vi "DB Tools Create Parameterized Query.vi"(4 "stored procedure? (F)":bool, 5 "auto-detect parameters? (F)":bool, 6 "error in (no error)":errorcluster, 7 "parameters":T3[](array[typedef]), 8 "SQL query":string, 9 "connection reference":T2) -> (0 "error out":errorcluster, 1 "parameters out":T3[](array[typedef]), 3 "command reference":T6)   [LabVIEW 2020, in "NI_Database_API.lvlib"]
doc: "Creates a parameterized <B>SQL query</B> and returns a <B>command reference</B> that you must free eventually. Unless you are detecting the parameters automatically, the number of elements in the <B>parameters</B> array must match the number of parameters you specify in <B>SQL query</B>. For stored procedures, set <B>stored procedure</B> to TRUE and <B>SQL query</B> to the name of the procedure you want to execute."
uses:
  <vilib>/addons/database/NI_Database_API.lvlib
  <vilib>/addons/database/Connection.llb/Conn ObjectReference.ctl
  <vilib>/addons/database/Command.llb/Cmd ObjectReference.ctl
  <vilib>/addons/database/Command.llb/Cmd DataMembers.ctl
  <vilib>/addons/database/Auxilliary.llb/DB Tools Parameter Info.ctl
  <vilib>/addons/database/Auxilliary.llb/DB Tools DataTypes.ctl
  <vilib>/addons/database/Auxilliary.llb/DB Tools Parameter Dir.ctl
  <vilib>/addons/database/Connection.llb/Conn Get Properties.vi
panel:
  in  "default":T1
  in  "default data":T1
  in  "ADODB._Command":refnum<k7>
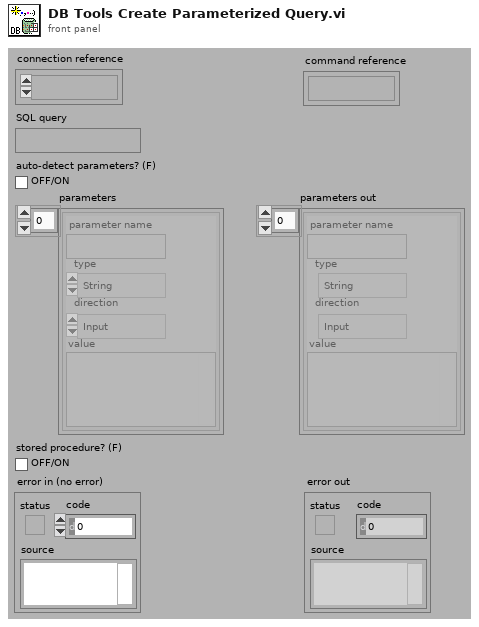
[diagram p1: front panel]
types:
  T1 = typedef "NI_Database_API.lvlib/Cmd DataMembers.ctl" = cluster{"ADODB._Command":refnum<k7>, "Connection":T2}
  T2 = typedef "NI_Database_API.lvlib/Conn ObjectReference.ctl" = refnum<k1>
  T3 = typedef "NI_Database_API.lvlib/DB Tools Parameter Info.ctl" = cluster{"parameter name":string, "type":T4, "direction":T5, "value":variant}
  T4 = typedef "NI_Database_API.lvlib/DB Tools DataTypes.ctl" = enum16{"String", "Long (I32)", "Single (SGL)", "Double (DBL)", "Date/Time", "Binary"}
  T5 = typedef "NI_Database_API.lvlib/DB Tools Parameter Dir.ctl" = enum32{"Input", "Output", "Input/Output", "Return Value"}
  T6 = typedef "NI_Database_API.lvlib/Cmd ObjectReference.ctl" = refnum<k1>
  T7 = typedef "NI_Database_API.lvlib/Conn Properties.ctl" = cluster{"command timeout (s)":i32, "connection string":string, "default database":string, "provider":string}
  T8 = typedef "NI_Database_API.lvlib/Conn DataMembers.ctl" = cluster{"ADODB._Connection":refnum<k7>, "recordset objects":i32, "command objects":i32}
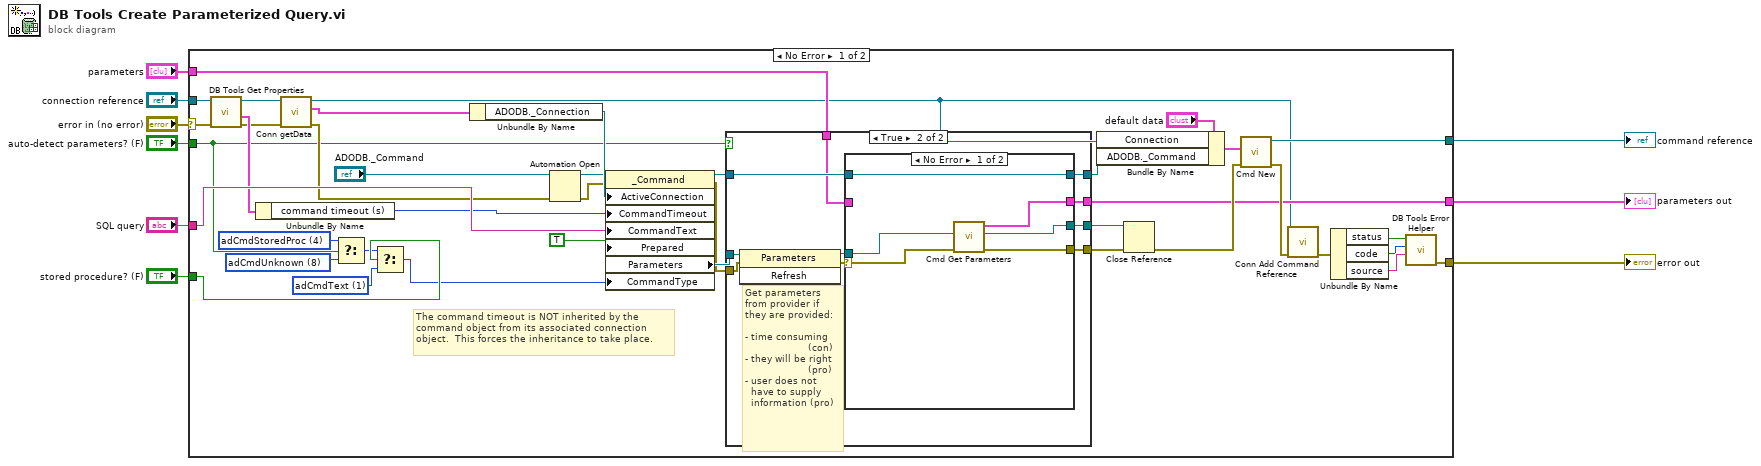
[diagram p0: block diagram]
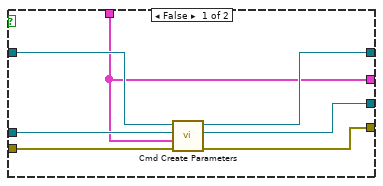
[diagram p2: hidden frame]
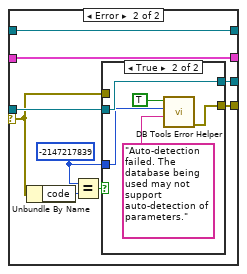
[diagram p3: hidden frame]
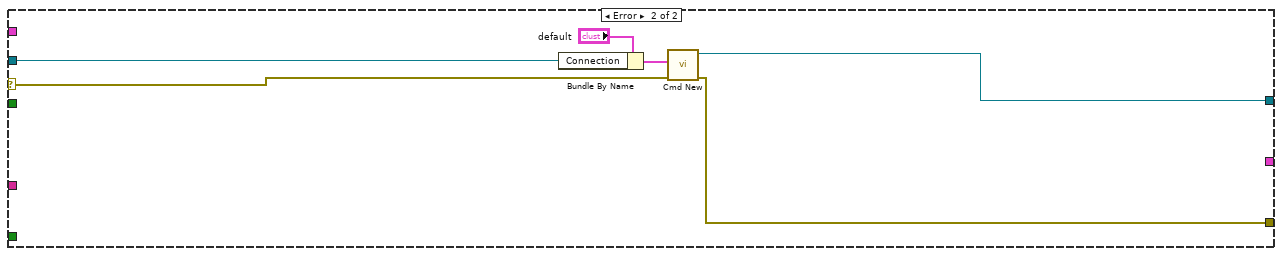
[diagram p5: hidden frame]
diagram:
  n1 = case shown="No Error" "error in (no error)" {
    selector: "error in (no error)" -> [w14 w92]
    tunnel: "stored procedure? (F)" -> [w49 _]
    tunnel: [w45 w89] -> w8
    tunnel: "auto-detect parameters? (F)" -> [w10 _]
    tunnel: "connection reference" -> [w38 w90]
    tunnel: "SQL query" -> [w37 _]
    tunnel: "parameters" -> [w31 _]
    tunnel: [w30 _] -> w3
    tunnel: [w20 w91] -> w2
    frame No Error {
      w11 = 8 items=["adCmdUnspecified"=-1, "adCmdUnknown"=8, "adCmdText"=1, "adCmdTable"=2, "adCmdStoredProc"=4, "adCmdFile"=256, "adCmdTableDirect"=512] ("CommandType")
      w48 = 1 items=["adCmdUnspecified"=-1, "adCmdUnknown"=8, "adCmdText"=1, "adCmdTable"=2, "adCmdStoredProc"=4, "adCmdFile"=256, "adCmdTableDirect"=512] ("CommandType")
      w12 = 4 items=["adCmdUnspecified"=-1, "adCmdUnknown"=8, "adCmdText"=1, "adCmdTable"=2, "adCmdStoredProc"=4, "adCmdFile"=256, "adCmdTableDirect"=512] ("CommandType")
      # "The command timeout is NOT inherited by the \ncommand object from its associated connection \nobject.  This forces the inheritance to take place."
      n2 = call-poly <vilib>:"DB Tools Get Properties.vi"("error in (no error)"=w14, "connection reference"=w38) -> ("error out"=w26:errorcluster, "connection properties"=w32:T7, "connection reference out"=w27:T2)  [unwired: 3 out]
      n3 = Unbundle By Name(w32) -> ("command timeout (s)"=w35:i32)
      n4 = call <vilib>:"Conn getData.vi"("error in (no error)"=w26, "connection reference"=w27) -> ("error out"=w16:errorcluster, "data"=w29:T8, "connection reference out"=w28:T2)  [unwired: 3 out]
      n5 = Select(t=w12, s=w10, f=w11) -> (s? t:f=w13:i32)
      n6 = Select(t=w13, s=w49, f=w48) -> (s? t:f=w34:i32)
      n7 = Unbundle By Name(w29) -> ("ADODB._Connection"=w25:refnum<k7>)
      n8 = Automation Open(error in (no error)=w16, Automation Refnum="ADODB._Command") -> (Automation Refnum=w17:refnum<k7>, error out=w19:errorcluster)  [unwired: 2 out]
      n9 = property class="_Command"(reference=w17, error in=w19, "ActiveConnection"=w25, "CommandTimeout"=w35, "CommandText"=w37, "Prepared"=TRUE, "CommandType"=w34) -> (reference out=w47:refnum<k7>, error out=w15:errorcluster, "Parameters"=w36:refnum<k7>)
      n10 = case shown="True" w10 {
        tunnel: w36 -> [w54 w66]
        tunnel: w15 -> [w55 w65]
        tunnel: w47 -> [w56 w63]
        tunnel: [w53 w59] -> w40
        tunnel: w31 -> [w51 w60]
        tunnel: [w52 w61] -> w42
        tunnel: [w51 w58] -> w30
        tunnel: [w50 w57] -> w41
        frame False {
          n11 = call <vilib>:"Cmd Create Parameters.vi"("error in (no error)"=w55, "parameters"=w51, "ADODB.Parameters"=w54, "ADODB._Command"=w56) -> ("error out"=w53:errorcluster, "ADODB.Parameters out"=w50:refnum<k7>, "ADODB._Command out"=w52:refnum<k7>)  [unwired: 1 out]
        }
        frame True {
          # "Get parameters \nfrom provider if\nthey are provided:\n\n- time consuming \n                     (con)\n- they will be right \n                     (pro)\n- user does not \n  have to supply\n  information (pro)"
          n12 = invoke class="Parameters" method="Refresh"(reference=w66, error in=w65) -> (reference out=w62:refnum<k7>, error out=w64:errorcluster)  [unwired: 1 in, 1 out]
          n13 = case shown="No Error" w64 {
            selector: w64 -> [w72 w79]
            tunnel: w63 -> [w71 w76]
            tunnel: w62 -> [w68 w80]
            tunnel: [w71 w76] -> w61
            tunnel: w60 -> [_ w77]
            tunnel: [w70 w78] -> w59
            tunnel: [w67 w77] -> w58
            tunnel: [w69 w75] -> w57
            frame No Error {
              n14 = call <vilib>:"Cmd Get Parameters.vi"("error in (no error)"=w72, "ADODB.Parameters"=w68) -> ("error out"=w70:errorcluster, "ADODB.Parameters out"=w69:refnum<k7>, "parameters"=w67:T3[])  [unwired: 1 in, 2 out]
            }
            frame Error {
              w73 = -2147217839
              n15 = Unbundle By Name(w79) -> ("code"=w74:i32)
              n16 = Equal?(x=w73, y=w74) -> (x = y?=w81:bool)
              n17 = case shown="True" w81 {
                tunnel: w80 -> [w82 w88]
                tunnel: w79 -> [w83 _]
                tunnel: [w83 w86] -> w78
                tunnel: [w82 w88] -> w75
                tunnel: w73 -> [_ w85]
                frame False {
                  # "some other error - \ndo nothing and \npass it through"
                }
                frame True {
                  n18 = call <vilib>:"DB Tools Error Helper.vi"("source"="Auto-detection failed. The database being used may not support auto-detection of parameters.", "code"=w85, "status"=TRUE) -> ("error out"=w86:errorcluster)  [unwired: 1 in, 7 out]
                }
              }
            }
          }
        }
      }
      n19 = Bundle By Name(cluster="default data", "Connection"=w28, "ADODB._Command"=w42) -> (w46:T1)
      n20 = Close Reference(reference=w41, error in (no error)=w40) -> (error out=w39:errorcluster)
      n21 = call <vilib>:"Cmd New.vi"("error in (no error)"=w39, "initial data"=w46) -> ("error out"=w43:errorcluster, "command reference"=w45:T6)  [unwired: 4 out]
      n22 = call <vilib>:"Conn Add Command Reference.vi"("error in (no error)"=w43, "connection reference"=w28) -> ("error out"=w21:errorcluster)  [unwired: 9 out]
      n23 = Unbundle By Name(w21) -> ("status"=w23:bool, "code"=w22:i32, "source"=w24:string)
      n24 = call <vilib>:"DB Tools Error Helper.vi"("source"=w24, "code"=w22, "status"=w23) -> ("error out"=w20:errorcluster)  [unwired: 1 in, 7 out]
    }
    frame Error {
      n25 = Bundle By Name(cluster="default", "Connection"=w90) -> (w94:T1)
      n26 = call <vilib>:"Cmd New.vi"("error in (no error)"=w92, "initial data"=w94) -> ("error out"=w91:errorcluster, "command reference"=w89:T6)  [unwired: 4 out]
    }
  }
  "command reference" <- w8
  "error out" <- w2
  "parameters out" <- w3
